vi "serial_04.vi"(0 "VISA resource name":refnum<visa-resource-name>="COM5") -> ()   [LabVIEW 2009]
doc: "The Basic Serial Read and Write example performs a Serial Port Read, a Serial Port Write, or a combination of these actions. The user selects the actions (read or write) on the front panel. If both are selected, the VI will write the data first, read data, and then close the VISA session that is opened to the port. This VI will wait until the specified number of bytes is received at the port. Only the number of bytes specified will be read.\n\nINSTRUCTIONS:\n1) Select the serial resource and configuration parameters (baud rate, data bits, parity, stop bits, flow control).\n2) Select the operations to be performed. \n3) Connect the serial port to your device. If no device is available, perform a loopback test by doing one of the following. Short pins 2 and 3 on a RS-232 cable or short pin 4 to pin 8 and pin 5 to pin 9 on a RS-485/422 cable. \n4) Run the VI to see the data read. (The \"read string\" will match the \"string to write\" if a loopback test was performed.)\n\nNote: The parameters set for the serial port must match the parameters of the connected instrument or device. In this example, the bytes to read parameter specifies the number of bytes that the serial port reads. If there were more bytes at the port than the number specified in bytes to read, those bytes would not be read. Also, if you specify to read more bytes than the number of bytes actually read, you might receive a timeout error message.\n\nOn the block diagram, the Configure Serial Port VI sets the configuration parameters. The front panel displays the controls used to configure the basic parameters, such as baud rate, data bits, and parity. Constants configure the other parameters the user probably does not need set. After the VISA Configure Serial Port VI opens the VISA session and configures the port, the VI passes the VISA resource name to other VIs that perform operations on that VISA resource. The VISA Write function sends a command to the serial device and the VISA Read function returns data based on the command. The VISA Close function then closes the reference to the serial device. It is important to close the reference; otherwise communication through with that port through protocols other than VISA might not be possible."
panel:
  in  "Start":bool=TRUE
  out "Meter":dbl(knob)=668.0 scale=0.0..1024.0
  out "Waveform Chart":i32(graph)=668
  # "Stop"
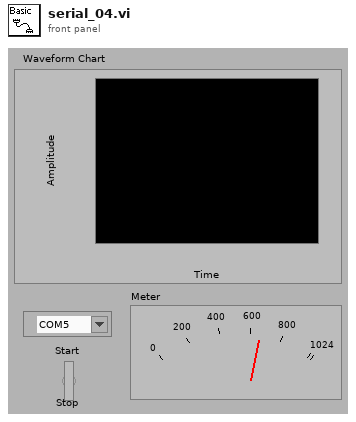
[diagram p1: front panel]
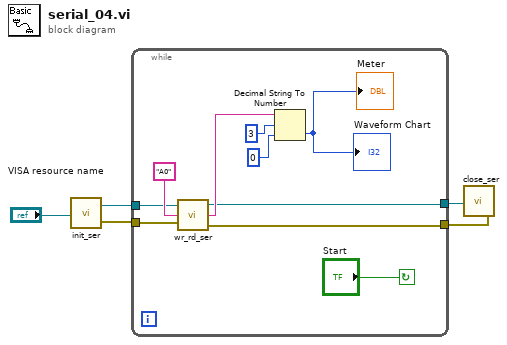
[diagram p0: block diagram]
diagram:
  n1 = call "init_ser.vi"("VISA resource name"="VISA resource name") -> ("VISA resource name out"=w3:refnum<visa-resource-name>, "error out"=w4:errorcluster)
  n2 = while {
    tunnel: w4 -> [w12]
    tunnel: w3 -> [w13]
    tunnel: [w6] -> w2
    tunnel: [w7] -> w1
    stop <- "Start" continue-if-true
    n3 = call "wr_rd_ser.vi"("error in"=w12, "string to write"="A0", "VISA resource name in"=w13) -> ("error out"=w6:errorcluster, "read buffer"=w11:string, "VISA resource name out"=w7:refnum<visa-resource-name>)
    n4 = Decimal String To Number(string=w11, offset=3, default (0L)=0) -> (number=→"Waveform Chart" →"Meter":i32)  [unwired: 1 out]
  }
  n5 = call "close_ser.vi"("error in"=w2, "VISA resource name in"=w1) -> ()
